vi "Init Logger.vi"(8 "error in (no error)":errorcluster, 10 "File Send Interval (Seconds)":dbl=600.0) -> (0 "error out":errorcluster, 3 "Logger out.lvclass":refnum<class "Logger.lvclass">)   [LabVIEW 2017, in "Logger.lvclass"]
uses:
  Logger.lvclass
  <vilib>/Skyline/Tag/Shared/typedefs/Tag Cluster Wrapper.ctl
  <vilib>/Skyline/Configuration/Configuration_class/NI Skyline Configuration.lvclass
  <vilib>/Skyline/Tag/Shared/typedefs/Tag Cluster.ctl
  <vilib>/Skyline/Tag/Shared/typedefs/DataType.ctl
  <vilib>/Skyline/Tag/Wrapper/Wrapper_class/NI Skyline Tag.lvclass
  Logger.lvclass/Logger.ctl
  <vilib>/Skyline/Tag/Wrapper/Wrapper AMQP_class/Query Tags AMQP.vi
  <vilib>/Skyline/Tag/Wrapper/Wrapper_class/Delete Tag (Multiple).vi
  <vilib>/Skyline/Tag/Wrapper/Wrapper AMQP_class/Open Tag AMQP.vi
  <vilib>/Skyline/Tag/Wrapper/Wrapper_class/Generate Tag Cluster (String).vi
  <vilib>/Skyline/Tag/Wrapper/Wrapper_class/Generate Tag Cluster (I32).vi
  <vilib>/Skyline/Message/sync/Open (Sync).vi
  <vilib>/Skyline/Message/NI Skyline Message (Sync).lvclass
  <vilib>/Skyline/Tag/Shared/NI Skyline Tag.lvlib
  <vilib>/Skyline/Tag/Wrapper/Wrapper AMQP_class/NI Skyline Tag AMQP.lvclass
  <vilib>/Skyline/Message/NI Skyline Message.lvclass
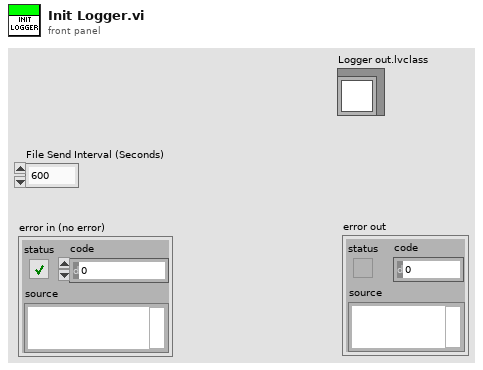
[diagram p1: front panel]
types:
  T1 = typedef "NI Skyline Tag.lvlib/Tag Cluster Wrapper.ctl" = cluster{"Configuration":refnum<class "NI Skyline Configuration.lvclass">, "Tag Cluster":T2}
  T2 = typedef "NI Skyline Tag.lvlib/Tag Cluster.ctl" = cluster{"Path":string, "Data Type":T3, "Value":variant, "Time Stamp":timestamp}
  T3 = typedef "NI Skyline Tag.lvlib/DataType.ctl" = enum32{"Double", "Integer", "String"}
  T4 = cluster{"Tag Units":string, "Tag Path":string, "Waveform":waveform(dbl), "Log":bool, "Tag Reference":refnum<class "NI Skyline Tag.lvclass">}
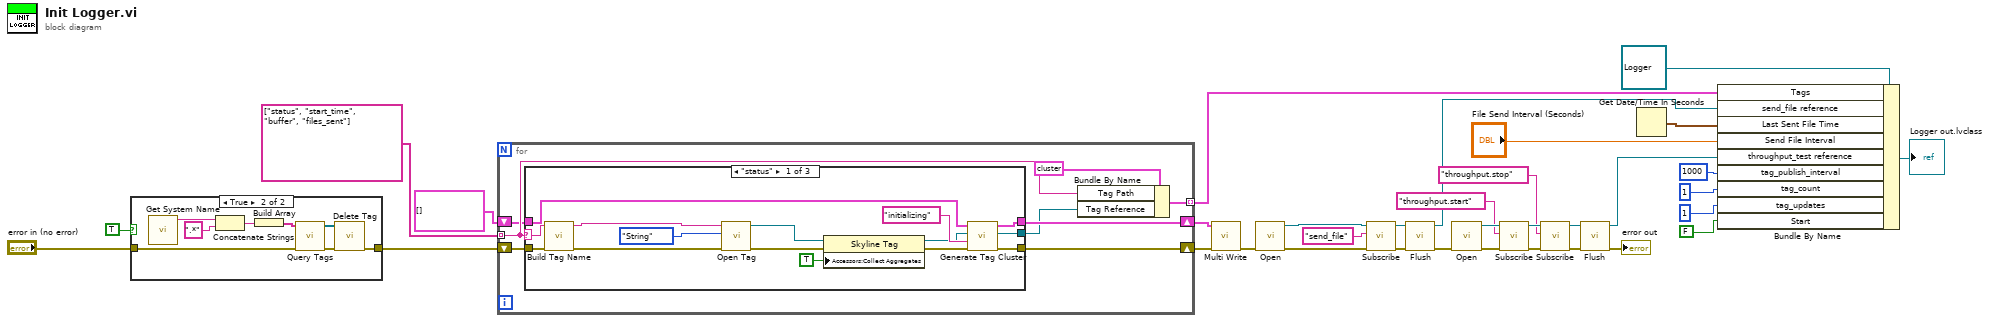
[diagram p0: block diagram]
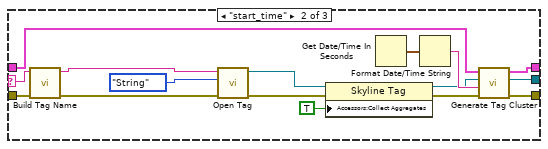
[diagram p3: hidden frame]
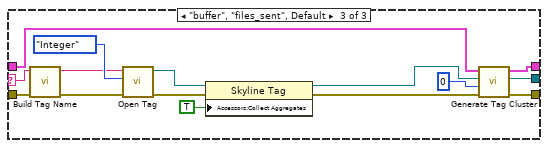
[diagram p4: hidden frame]
diagram:
  n1 = case shown="True" TRUE {
    tunnel: "error in (no error)" -> [w35 w37]
    tunnel: [w35 w36] -> w2
    frame False {
    }
    frame True {
      n2 = call "Get System Name.vi"() -> ("name"=w41:string)  [unwired: 11 in]
      n3 = Concatenate Strings(w41, ".*" ("string")) -> (w39:string)
      n4 = Build Array(w39) -> (w38:string[])
      n5 = call-poly <vilib>:"Query Tags.vi"("error in (no error)"=w37, "paths (*)"=w38) -> ("error out"=w43:errorcluster, "tags"=w42:refnum<class "NI Skyline Tag.lvclass">[])  [unwired: 8 in]
      n6 = call-poly <vilib>:"Delete Tag.vi"("error in (no error)"=w43, "tags in"=w42) -> ("error out"=w36:errorcluster)  [unwired: 9 in]
    }
  }
  n7 = for {
    shift-right: [w51] -> w7
    shift-left: w2 -> [w48]
    tunnel: string[] ["status", "start_time", "buffer", "files_sent"] -> [w49] mode=indexing
    tunnel: [w50] -> w28 mode=indexing
    shift-right: [w47] -> w5
    shift-left: T1[] [] ("tag clusters out") -> [w46]
    n8 = case shown="\"status\"" w49 {
      selector: w49 -> [w65 w81 w96]
      tunnel: [w63 w75 w93] -> w51
      tunnel: [w64 w76 w94] -> w44
      tunnel: w48 -> [w66 w80 w97]
      tunnel: [w59 w73 w89] -> w47
      tunnel: w46 -> [w57 w74 w88]
      frame "status" {
        n9 = call "Build Tag Name.vi"("error in (no error)"=w66, "Tag"=w65) -> ("error out"=w62:errorcluster, "System Tag"=w61:string)  [unwired: 8 in]
        n10 = call-poly <vilib>:"Open Tag.vi"("error in (no error)"=w62, "data type"=DataType."String" ("Data Type"), "path"=w61) -> ("error out"=w54:errorcluster, "tag out"=w55:refnum<class "NI Skyline Tag.lvclass">)  [unwired: 7 in]
        n11 = property on="Property Node" class="Skyline Tag"(reference=w55, error in=w54, "Accessors:Collect Aggregates"=TRUE ("Collect Aggregates")) -> (reference out=w53:refnum<class "NI Skyline Tag.lvclass">, error out=w52:errorcluster)
        n12 = call-poly <vilib>:"Generate Tag Cluster.vi"("error in (no error)"=w52, "value"="initializing" ("string"), "tag in"=w53, "tag clusters in"=w57) -> ("error out"=w63:errorcluster, "tag out"=w64:refnum<class "NI Skyline Tag.lvclass">, "tag clusters out"=w59:T1[])  [unwired: 5 in]
      }
      frame "start_time" {
        n13 = call "Build Tag Name.vi"("error in (no error)"=w80, "Tag"=w81) -> ("error out"=w77:errorcluster, "System Tag"=w78:string)  [unwired: 8 in]
        n14 = call-poly <vilib>:"Open Tag.vi"("error in (no error)"=w77, "data type"=DataType."String" ("Data Type"), "path"=w78) -> ("error out"=w69:errorcluster, "tag out"=w70:refnum<class "NI Skyline Tag.lvclass">)  [unwired: 7 in]
        n15 = property on="Property Node" class="Skyline Tag"(reference=w70, error in=w69, "Accessors:Collect Aggregates"=TRUE ("Collect Aggregates")) -> (reference out=w68:refnum<class "NI Skyline Tag.lvclass">, error out=w67:errorcluster)
        n16 = Get Date/Time In Seconds() -> (seconds since 1Jan1904=w82:timestamp)
        n17 = Format Date/Time String(seconds (now)=w82) -> (date/time string=w72:string)  [unwired: 2 in]
        n18 = call-poly <vilib>:"Generate Tag Cluster.vi"("error in (no error)"=w67, "value"=w72, "tag in"=w68, "tag clusters in"=w74) -> ("error out"=w75:errorcluster, "tag out"=w76:refnum<class "NI Skyline Tag.lvclass">, "tag clusters out"=w73:T1[])  [unwired: 5 in]
      }
      frame "buffer", "files_sent", Default {
        n19 = call "Build Tag Name.vi"("error in (no error)"=w97, "Tag"=w96) -> ("error out"=w91:errorcluster, "System Tag"=w90:string)  [unwired: 8 in]
        n20 = call-poly <vilib>:"Open Tag.vi"("error in (no error)"=w91, "data type"=DataType."Integer" ("Data Type"), "path"=w90) -> ("error out"=w86:errorcluster, "tag out"=w87:refnum<class "NI Skyline Tag.lvclass">)  [unwired: 7 in]
        n21 = property on="Property Node" class="Skyline Tag"(reference=w87, error in=w86, "Accessors:Collect Aggregates"=TRUE ("Collect Aggregates")) -> (reference out=w84:refnum<class "NI Skyline Tag.lvclass">, error out=w83:errorcluster)
        n22 = call-poly <vilib>:"Generate Tag Cluster.vi"("error in (no error)"=w83, "value"=0, "tag in"=w84, "tag clusters in"=w88) -> ("error out"=w93:errorcluster, "tag out"=w94:refnum<class "NI Skyline Tag.lvclass">, "tag clusters out"=w89:T1[])  [unwired: 5 in]
      }
    }
    n23 = Bundle By Name(cluster=T4 {"Tag Units"="", "Tag Path"="", "Waveform"={"t0"=timestamp(0 s since 1904-01-01), "dt"=1.0, "Y"=[]}, "Log"=FALSE, "Tag Reference"=refnum} ("Tag"), "Tag Path"=w49, "Tag Reference"=w44) -> (w50:T4)
  }
  n24 = call <vilib>:"Multi Write.vi"("error in (no error)"=w7, "tag clusters"=w5) -> ("error out"=w6:errorcluster)  [unwired: 9 in]
  n25 = call-poly <vilib>:"Open.vi"("error in (no error)"=w6) -> ("error out"=w31:errorcluster, "message sync out"=w32:refnum<class "NI Skyline Message (Sync).lvclass">)  [unwired: 9 in]
  n26 = call-dynamic "Subscribe.vi"("error in (no error)"=w31, "topic"="send_file" ("Tag"), "message sync in"=w32) -> ("error out"=w25:errorcluster, "message sync out"=w24:refnum<class "NI Skyline Message (Sync).lvclass">)  [unwired: 7 in]
  n27 = call <vilib>:"Flush.vi"("error in (no error)"=w25, "message sync in"=w24) -> ("error out"=w20:errorcluster, "message sync out"=w10:refnum<class "NI Skyline Message (Sync).lvclass">)  [unwired: 8 in]
  n28 = call-poly <vilib>:"Open.vi"("error in (no error)"=w20) -> ("error out"=w23:errorcluster, "message sync out"=w22:refnum<class "NI Skyline Message (Sync).lvclass">)  [unwired: 9 in]
  n29 = call-dynamic "Subscribe.vi"("error in (no error)"=w23, "topic"="throughput.start", "message sync in"=w22) -> ("error out"=w15:errorcluster, "message sync out"=w14:refnum<class "NI Skyline Message (Sync).lvclass">)  [unwired: 7 in]
  n30 = call-dynamic "Subscribe.vi"("error in (no error)"=w15, "topic"="throughput.stop", "message sync in"=w14) -> ("error out"=w12:errorcluster, "message sync out"=w13:refnum<class "NI Skyline Message (Sync).lvclass">)  [unwired: 7 in]
  n31 = call <vilib>:"Flush.vi"("error in (no error)"=w12, "message sync in"=w13) -> ("error out"=→"error out":errorcluster, "message sync out"=w9:refnum<class "NI Skyline Message (Sync).lvclass">)  [unwired: 8 in]
  n32 = Get Date/Time In Seconds() -> (seconds since 1Jan1904=w29:timestamp)
  n33 = Bundle By Name(cluster=refnum<class "Logger.lvclass"> refnum ("Logger out.lvclass"), "Tags"=w28, "send_file reference"=w10, "Last Sent File Time"=w29, "Send File Interval"="File Send Interval (Seconds)", "throughput_test reference"=w9, "tag_publish_interval"=1000, "tag_count"=1, "tag_updates"=1, "Start"=FALSE) -> (→"Logger out.lvclass":refnum<class "Logger.lvclass">)
